vi "tcpclient.vi"() -> ()   [LabVIEW 2021]
panel:
  out "Waveform Graph":dbl[](graph)
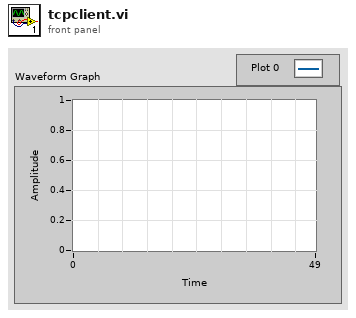
[diagram p1: front panel]
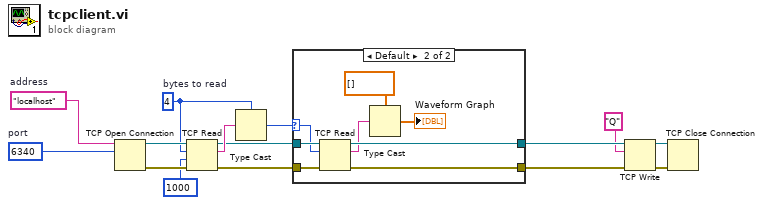
[diagram p0: block diagram]
diagram:
  w3 = 4  # bytes to read
  w7 = u16 6340  # port
  w8 = "localhost"  # address
  n1 = TCP Open Connection(address=w8, remote port or service name=w7) -> (connection ID=w15:refnum<k5>, error out=w14:errorcluster)  [unwired: 3 in]
  n2 = TCP Read(connection ID=w15, bytes to read=w3, error in (no error)=w14, 9:1000 ("timeout ms (25000)")) -> (connection ID out=w5:refnum<k5>, data out=w6:string, error out=w4:errorcluster)  [unwired: 1 in]
  n3 = Type Cast(type=w3, x=w6) -> (*(type *) &x=w2:i32)
  n4 = case shown="Default" w2 {
    selector: w2 -> [_ w18]
    tunnel: w5 -> [w17 w25]
    tunnel: w4 -> [w16 w24]
    tunnel: [w17 w21] -> w12
    tunnel: [w16 w20] -> w10
    frame ..0 {
      # "The server has not written any data"
    }
    frame Default {
      n5 = TCP Read(connection ID=w25, bytes to read=w18, error in (no error)=w24) -> (connection ID out=w21:refnum<k5>, data out=w19:string, error out=w20:errorcluster)  [unwired: 2 in]
      n6 = Type Cast(type=dbl[] [] ("chart"), x=w19) -> (*(type *) &x=→"Waveform Graph":dbl[])
    }
  }
  n7 = TCP Write(connection ID=w12, data in="Q", error in (no error)=w10) -> (connection ID out=w13:refnum<k5>, error out=w11:errorcluster)  [unwired: 2 out]
  n8 = TCP Close Connection(connection ID=w13, error in (no error)=w11) -> ()  [unwired: 1 in, 2 out]
